vi "Class to Variant.vi"(8 "error in (no error)":errorcluster, 10 "Data in":variant, 11 "VIPC Apply Node in":refnum<class "VIPC Apply Node.lvclass">) -> (0 "error out":errorcluster, 1 "Serialized Object Name":string, 2 "Data Out":variant, 3 "VIPC Apply Node out":refnum<class "VIPC Apply Node.lvclass">)   [LabVIEW 2014, in "VIPC Apply Node.lvclass"]
uses:
  VIPC Apply Node.lvclass
  Shared/Controls/VIPC Apply - STYP.ctl
  VIPC Apply Node.lvclass/VIPC Apply Node.ctl
  Classes/Build Job/Build Job.lvclass
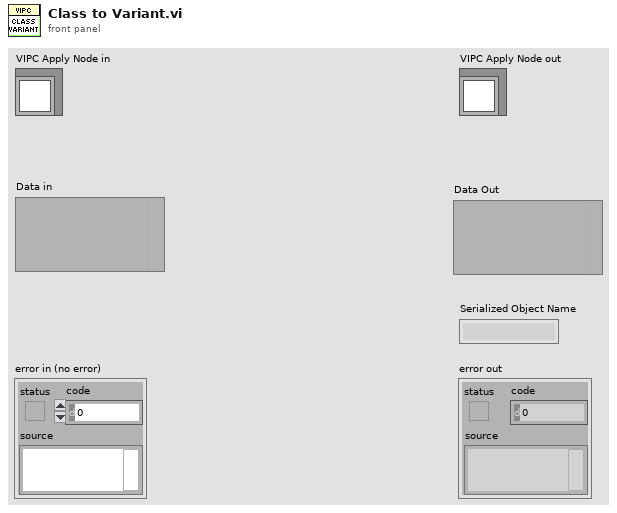
[diagram p1: front panel]
types:
  T1 = typedef "VIPC Apply - STYP.ctl" = cluster{"VIPC Path":string, "LabVIEW Version":string}
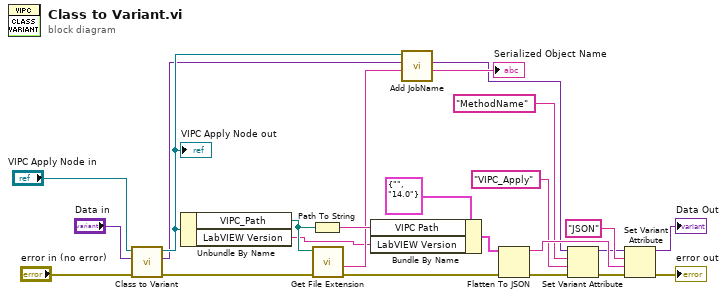
[diagram p0: block diagram]
diagram:
  n1 = call-parent "Class to Variant.vi"("error in (no error)"="error in (no error)", "Data in"="Data in", "Build Job in"="VIPC Apply Node in") -> ("error out"=w6:errorcluster, "Data Out"=w3:variant, "Build Job out"=w8:refnum<class "VIPC Apply Node.lvclass">)  [unwired: 5 in, 1 out]
  "VIPC Apply Node out" <- w8
  n2 = Unbundle By Name(w8) -> ("VIPC_Path"=w7:path, "LabVIEW Version"=w1:string)
  n3 = Path To String(path=w7) -> (string=w13:string)
  n4 = call <vilib>:"Get File Extension.vi"("error in (no error)"=w6, "file"=w7) -> ("error out"=w5:errorcluster, "filename without extension"=w9:string)  [unwired: 6 in, 2 out]
  n5 = Bundle By Name(cluster=T1 {"VIPC Path"="", "LabVIEW Version"="14.0"} ("VIPC Apply"), "VIPC Path"=w13, "LabVIEW Version"=w1) -> (w15:T1)
  n6 = call "Add JobName.vi"("Job Target"=w9, "Data in"=w3, "Build Job in"=w8) -> ("Job Name"=→"Serialized Object Name":string, "Data Out"=w2:variant)  [unwired: 7 in]
  n7 = Flatten To JSON(anything=w15, error in (no error)=w5) -> (JSON string=w20:string, 11:w21:errorcluster)  [unwired: 1 in]
  n8 = Set Variant Attribute(Variant=w2, name="MethodName", value="VIPC_Apply", error in=w21) -> (Variant out=w10:variant, error out=w16:errorcluster)  [unwired: 1 out]
  n9 = Set Variant Attribute(Variant=w10, name="JSON" ("Name"), value=w20, error in=w16) -> (Variant out=→"Data Out":variant, error out=→"error out":errorcluster)  [unwired: 1 out]
